vi "Trigger the captured image.vi"() -> ()   [LabVIEW 2009]
uses:
  D/Program Files (x86)/National Instruments/LabVIEW 2015/user.lib/LabViewDVPCamera/LabViewDVPCamera.lvlib
panel:
  in  "Trigger":bool
  in  "CloseFlg":i32
  out "handle":u32
  out "new picture":picture caption="新图片"
  in  "CameraList":u16(ring) items=["USB2_1.2M_MONO(39)@UE121000027", "USB2_3M(19)@1112121"]
  in  "Set":bool
  in  "Close":bool
  in  "Open":bool
  in  "ScanCamera":bool
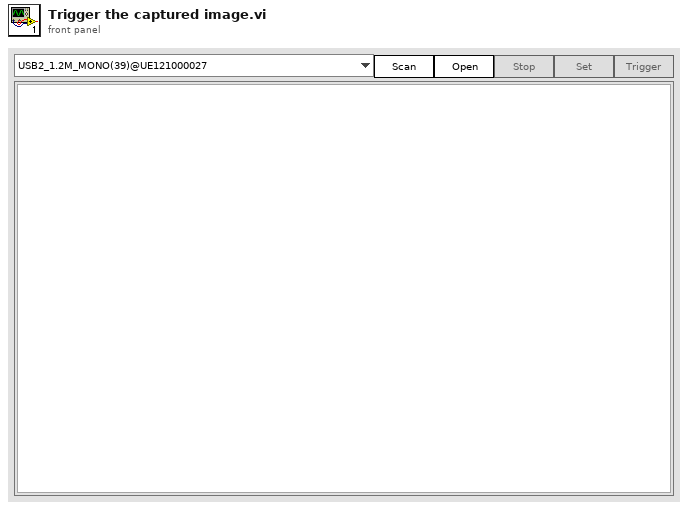
[diagram p1: front panel]
types:
  T1 = enum8{"Enabled", "Disabled", "Disabled and Grayed Out"}
  T2 = typedef "LVStringsAndValuesArrayTypeDef_U16.ctl" = cluster{"String":string, "Value":u16}[]
  T3 = cluster{"image type":i16, "image depth":u8, u8[], "无符号8位数组":u8[], u32[], cluster{u16, u16, u16, u16}}
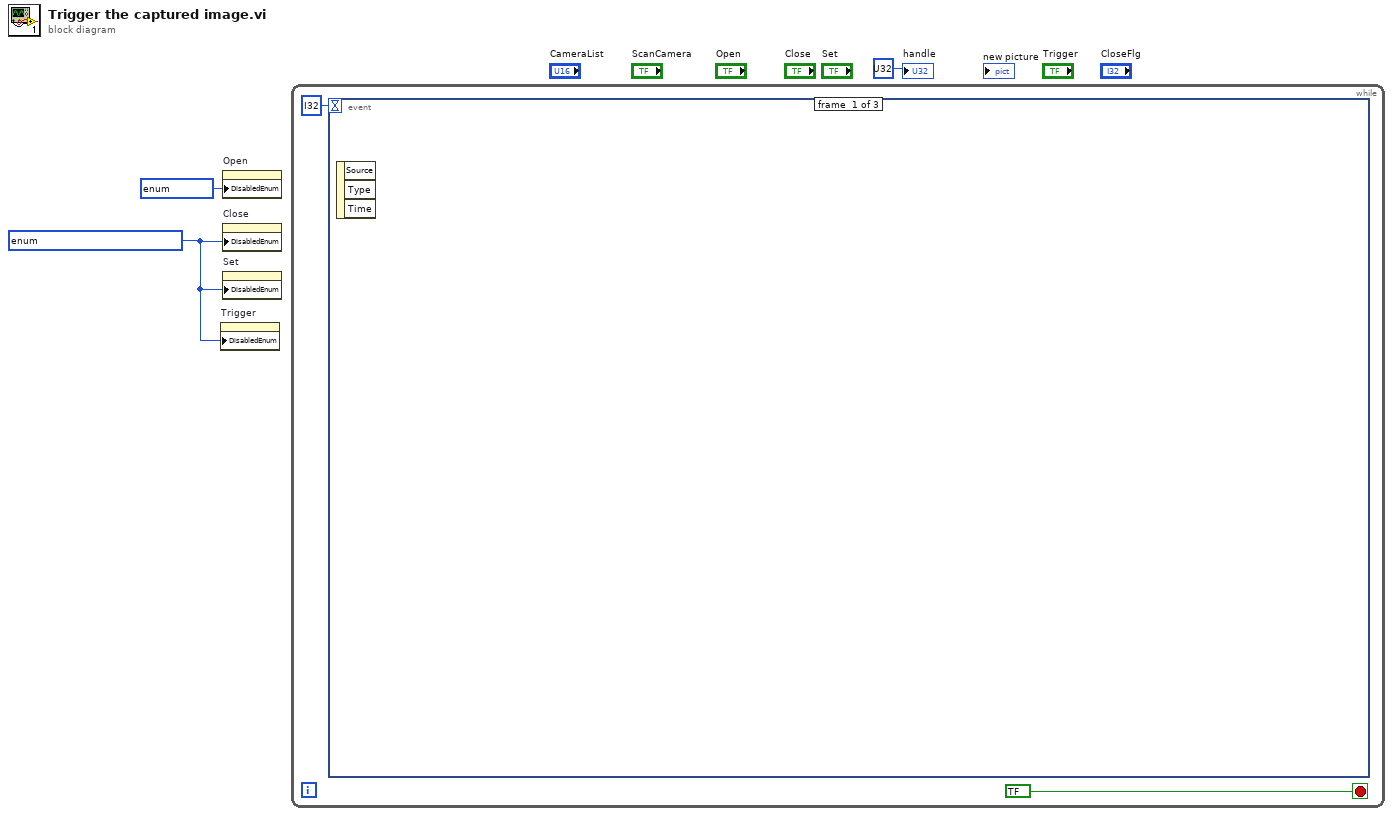
[diagram p0: block diagram]
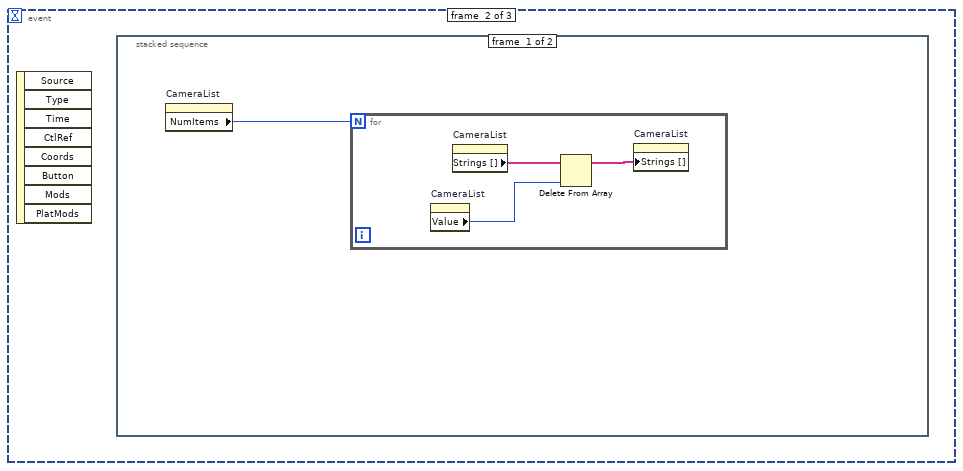
[diagram p2: hidden frame]
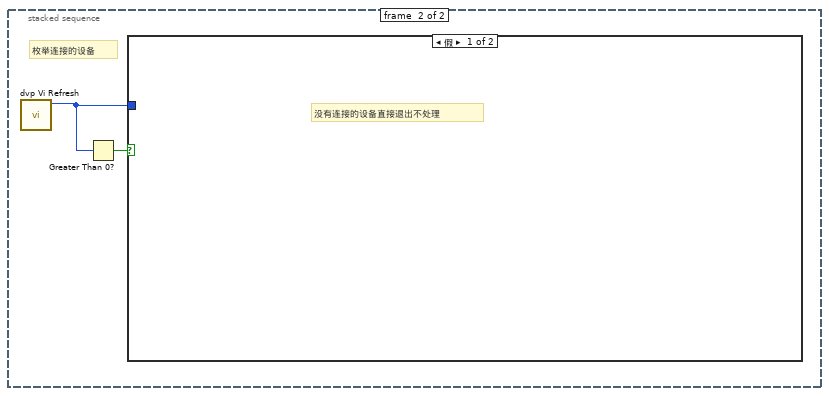
[diagram p3: hidden frame]
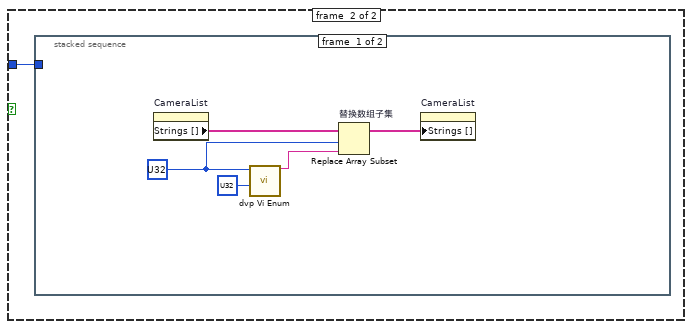
[diagram p4: hidden frame]
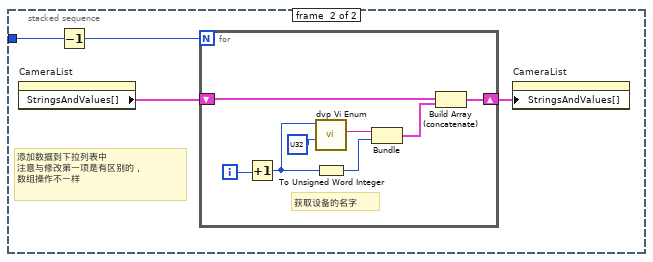
[diagram p5: hidden frame]
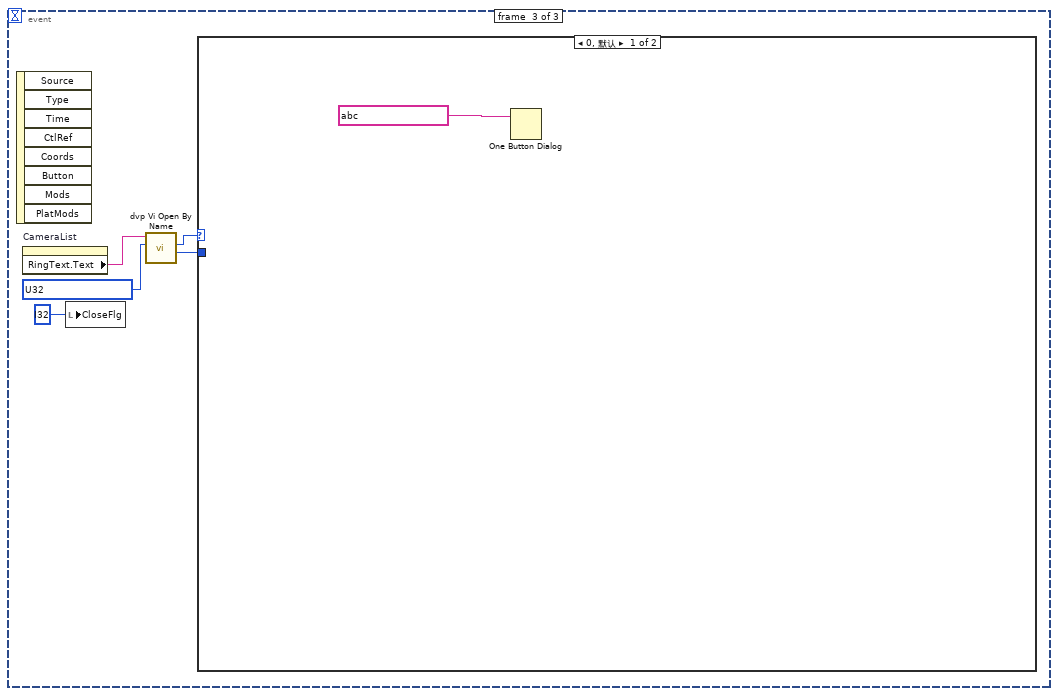
[diagram p6: hidden frame]
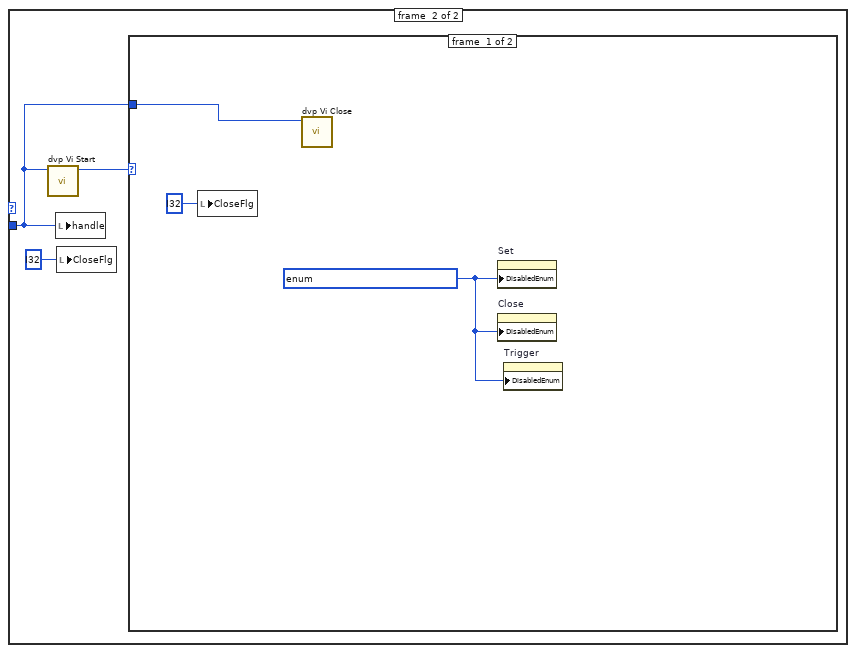
[diagram p7: hidden frame]
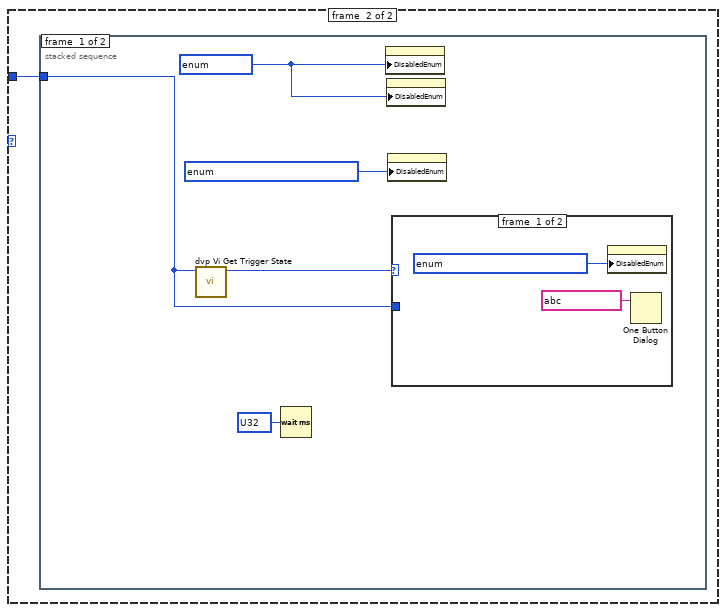
[diagram p8: hidden frame]
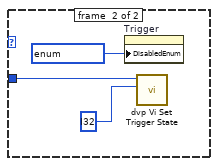
[diagram p9: hidden frame]
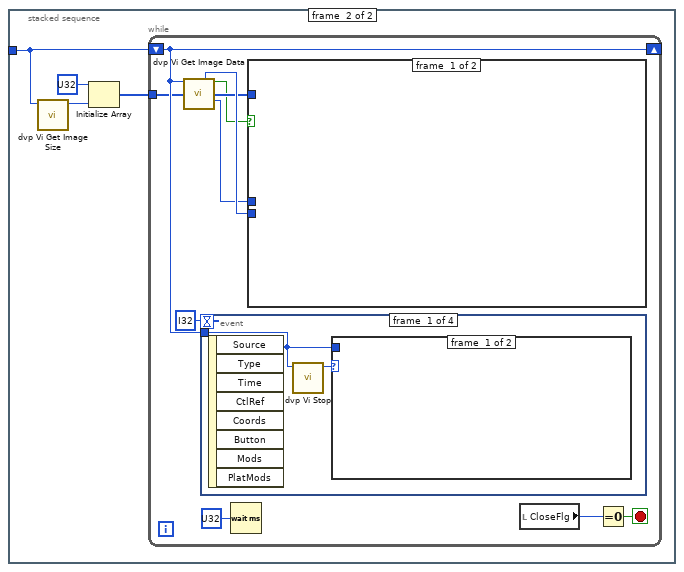
[diagram p10: hidden frame]
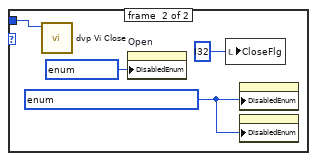
[diagram p11: hidden frame]
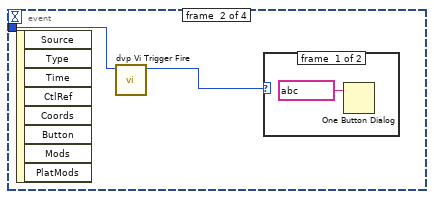
[diagram p12: hidden frame]
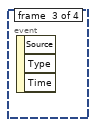
[diagram p14: hidden frame]
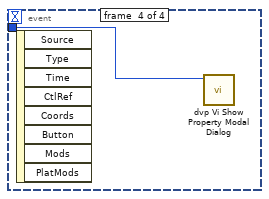
[diagram p15: hidden frame]
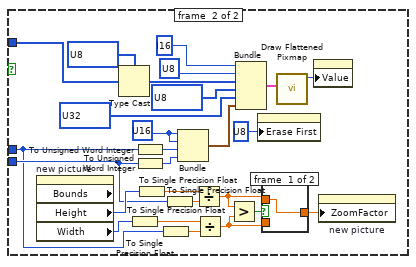
[diagram p16: hidden frame]
diagram:
  w1 = T1 ? ("禁用")
  n1 = property on="Trigger" class="Bool"("DisabledEnum"=w1) -> ()  [unwired: 2 in, 2 out]
  n2 = property on="Open" class="Bool"("DisabledEnum"=T1 ? ("禁用")) -> ()  [unwired: 2 in, 2 out]
  n3 = property on="Close" class="Bool"("DisabledEnum"=w1) -> ()  [unwired: 2 in, 2 out]
  n4 = property on="Set" class="Bool"("DisabledEnum"=w1) -> ()  [unwired: 2 in, 2 out]
  n5 = while {
    stop <- bool ? stop-if-true
    n6 = event shown="[2] \"Open\": 鼠标按下" {
      selector: _ -> [_ _ _]
      dyn-events: _ -> [_ _ _]
      timeout: i32 ? -> [_ _ _]
      event #0 {
        n7 = event-data() -> ()  [unwired: 1 in, 3 out]
      }
      event #1 {
        n8 = event-data() -> ()  [unwired: 1 in, 8 out]
        n9 = stacked-sequence "清除下拉列表的数据" {
          frame #0 {
            n10 = property on="CameraList" class="Ring (严格)"() -> ("NumItems"=w6:u32)  [unwired: 2 in, 2 out]
            n11 = for {
              N: w6 -> [_]
              n12 = property on="CameraList" class="Ring (严格)"() -> ("Value"=w8:u16)  [unwired: 2 in, 2 out]
              n13 = property on="CameraList" class="Ring (严格)"() -> ("Strings []"=w7:string[])  [unwired: 2 in, 2 out]
              n14 = Delete From Array ("删除数组元素")(array=w7, index=w8) -> (array with subset deleted=w9:string[])  [unwired: 1 in, 1 out]
              n15 = property on="CameraList" class="Ring (严格)"("Strings []"=w9) -> ()  [unwired: 2 in, 2 out]
            }
          }
          frame #1 {
            # "枚举连接的设备"
            n16 = call "dvp Vi Refresh.vi"() -> ("pCount out"=w11:u32)  [unwired: 10 in, 1 out]
            n17 = Greater Than 0?(x=w11) -> (x > 0?=w10:bool)
            n18 = case shown="假" w10 {
              tunnel: w11 -> [_ w12]
              frame #0 {
                # "没有连接的设备直接退出不处理"
              }
              frame #1 {
                n19 = stacked-sequence {
                  tunnel: w12 -> [_ w19]
                  frame #0 {
                    w13 = u32 ? ("index")
                    n20 = property on="CameraList" class="Ring (严格)"() -> ("Strings []"=w16:string[])  [unwired: 2 in, 2 out]
                    n21 = call "dvp Vi Enum.vi"("unSize"=u32 ?, "index"=w13) -> ("friendlyName out"=w15:string)  [unwired: 8 in, 1 out]
                    n22 = Replace Array Subset "替换数组子集"(array=w16, new element=w15, index=w13) -> (w17:string[])
                    n23 = property on="CameraList" class="Ring (严格)"("Strings []"=w17) -> ()  [unwired: 2 in, 2 out]
                  }
                  frame #1 {
                    # "添加数据到下拉列表中\n注意与修改第一项是有区别的，\n数组操作不一样"
                    n24 = property on="CameraList" class="Ring (严格)"() -> ("StringsAndValues[]"=w21:T2)  [unwired: 2 in, 2 out]
                    n25 = Decrement(x=w19) -> (x-1=w18:u32)
                    n26 = for {
                      N: w18 -> [_]
                      shift-right: [w28] -> w20
                      shift-left: w21 -> [w26]
                      i -> [w23]
                      # "获取设备的名字"
                      n27 = Increment(x=w23) -> (x+1=w22:i32)
                      n28 = call "dvp Vi Enum.vi"("unSize"=u32 ?, "index"=w22) -> ("friendlyName out"=w29:string)  [unwired: 8 in, 1 out]
                      n29 = To Unsigned Word Integer(number=w22) -> (unsigned 16bit integer=w25:u16)
                      n30 = Bundle("friendlyName out"=w29, w25) -> (w27:cluster{"friendlyName out":string, u16})  [unwired: 1 in]
                      n31 = Build Array (concatenate)(w26, w27) -> (w28:T2)
                    }
                    n32 = property on="CameraList" class="Ring (严格)"("StringsAndValues[]"=w20) -> ()  [unwired: 2 in, 2 out]
                  }
                }
              }
            }
          }
        }
      }
      event #2 {
        w32 = u32 ? items=["OPEN_OFFLINE", "OPEN_NORMAL"] ("type")
        n33 = event-data() -> ()  [unwired: 1 in, 8 out]
        n34 = property on="CameraList" class="Ring (严格)"() -> ("RingText.Text"=w31:string)  [unwired: 2 in, 2 out]
        n35 = local write "CloseFlg"(i32 ? ("CloseFlg")) -> ()
        n36 = call "dvp Vi Open By Name.vi"("type"=w32, "friendlyName"=w31) -> ("pHandle out"=w34:u32, "function return"=w33:u32)  [unwired: 7 in, 1 out]
        n37 = case shown="0, 默认" w33 {
          tunnel: w34 -> [_ w38]
          frame #0 {
            n38 = One Button Dialog(message=string ? ("消息")) -> ()  [unwired: 1 in, 1 out]
          }
          frame #1 {
            n39 = call "dvp Vi Start.vi"("handle"=w38) -> ("function return"=w36:u32)  [unwired: 10 in]
            n40 = local write "handle"(w38) -> ()
            n41 = local write "CloseFlg"(i32 ? ("CloseFlg")) -> ()
            n42 = case shown="1" w36 {
              tunnel: w38 -> [w41 w42]
              frame #0 {
                w39 = T1 ? ("禁用")
                n43 = local write "CloseFlg"(i32 ? ("CloseFlg")) -> ()
                n44 = call "dvp Vi Close.vi"("handle"=w41) -> ()  [unwired: 10 in, 1 out]
                n45 = property on="Set" class="Bool"("DisabledEnum"=w39) -> ()  [unwired: 2 in, 2 out]
                n46 = property on="Close" class="Bool"("DisabledEnum"=w39) -> ()  [unwired: 2 in, 2 out]
                n47 = property on="Trigger" class="Bool"("DisabledEnum"=w39) -> ()  [unwired: 2 in, 2 out]
              }
              frame #1 {
                n48 = stacked-sequence {
                  tunnel: w42 -> [w44 w54]
                  frame #0 {
                    w46 = T1 ? ("禁用")
                    n49 = call "dvp Vi Get Trigger State.vi"("handle"=w44) -> ("function return"=w45:u32)  [unwired: 9 in, 1 out]
                    n50 = Wait (ms)(milliseconds to wait=u32 ? ("等待时间（毫秒）")) -> ()  [unwired: 1 out]
                    n51 = property on="Set" class="Bool"("DisabledEnum"=w46) -> ()  [unwired: 2 in, 2 out]
                    n52 = property on="Close" class="Bool"("DisabledEnum"=w46) -> ()  [unwired: 2 in, 2 out]
                    n53 = property on="Open" class="Bool"("DisabledEnum"=T1 ? ("禁用")) -> ()  [unwired: 2 in, 2 out]
                    n54 = case shown="1" w45 {
                      tunnel: w44 -> [_ w51]
                      frame #0 {
                        n55 = property on="Trigger" class="Bool"("DisabledEnum"=T1 ? ("禁用")) -> ()  [unwired: 2 in, 2 out]
                        n56 = One Button Dialog(message=string ? ("消息")) -> ()  [unwired: 1 in, 1 out]
                      }
                      frame #1 {
                        n57 = property on="Trigger" class="Bool"("DisabledEnum"=T1 ? ("禁用")) -> ()  [unwired: 2 in, 2 out]
                        n58 = call "dvp Vi Set Trigger State.vi"("TriggerState"=i32 ?, "handle"=w51) -> ()  [unwired: 9 in, 1 out]
                      }
                    }
                  }
                  frame #1 {
                    n59 = call "dvp Vi Get Image Size.vi"("handle"=w54) -> ("function return"=w55:u32)  [unwired: 10 in]
                    n60 = Initialize Array(u32 ? ("元素"), w55) -> (w53:u32[])
                    n61 = while {
                      shift-right: [w62] -> _
                      shift-left: w54 -> [w62]
                      tunnel: w53 -> [w61]
                      stop <- w65 stop-if-true
                      n62 = call "dvp Vi Get Image Data.vi"("handle"=w62, "pbuffer"=w61) -> ("piHeight out"=w60:i32, "function return"=w57:bool, "pbuffer out"=w58:u32[], "piWidth out"=w59:i32)  [unwired: 9 in, 1 out]
                      n63 = event shown="[3] \"Set\": 鼠标按下" {
                        selector: _ -> [_ _ _ _]
                        dyn-events: _ -> [_ _ _ _]
                        timeout: i32 ? -> [_ _ _ _]
                        tunnel: w62 -> [w67 w74 _ w76]
                        event #0 {
                          n64 = event-data() -> ()  [unwired: 1 in, 8 out]
                          n65 = call "dvp Vi Stop.vi"("handle"=w67) -> ("function return"=w68:u32)  [unwired: 10 in]
                          n66 = case shown="1" w68 {
                            tunnel: w67 -> [_ w70]
                            frame #0 {
                            }
                            frame #1 {
                              w69 = T1 ? ("禁用")
                              n67 = call "dvp Vi Close.vi"("handle"=w70) -> ()  [unwired: 10 in, 1 out]
                              n68 = property on="Open" class="Bool"("DisabledEnum"=T1 ? ("禁用")) -> ()  [unwired: 2 in, 2 out]
                              n69 = local write "CloseFlg"(i32 ? ("CloseFlg")) -> ()
                              n70 = property on="Close" class="Bool"("DisabledEnum"=w69) -> ()  [unwired: 2 in, 2 out]
                              n71 = property on="Set" class="Bool"("DisabledEnum"=w69) -> ()  [unwired: 2 in, 2 out]
                            }
                          }
                        }
                        event #1 {
                          n72 = event-data() -> ()  [unwired: 1 in, 8 out]
                          n73 = call "dvp Vi Trigger Fire.vi"("handle"=w74) -> ("function return"=w73:u32)  [unwired: 10 in]
                          n74 = case shown="1" w73 {
                            frame #0 {
                              n75 = One Button Dialog(message=string ? ("消息")) -> ()  [unwired: 1 in, 1 out]
                            }
                            frame #1 {
                            }
                          }
                        }
                        event #2 {
                          n76 = event-data() -> ()  [unwired: 1 in, 3 out]
                        }
                        event #3 {
                          n77 = event-data() -> ()  [unwired: 1 in, 8 out]
                          n78 = call "dvp Vi Show Property Modal Dialog.vi"("handle"=w76) -> ()  [unwired: 10 in, 1 out]
                        }
                      }
                      n79 = Wait (ms)(milliseconds to wait=u32 ? ("等待时间（毫秒）")) -> ()  [unwired: 1 out]
                      n80 = case shown="真" w57 {
                        tunnel: w59 -> [_ w77]
                        tunnel: w60 -> [_ w78]
                        tunnel: w58 -> [_ w79]
                        frame #0 {
                        }
                        frame #1 {
                          w99 = u16 ?
                          n81 = property on="new picture" class="Pict" props=[]() -> ("Height"=w94:u32, "Width"=w93:u32)  [unwired: 2 in, 3 out]
                          n82 = Type Cast(type=u8[] ?, x=w79) -> (*(type *) &x=w83:u8[])
                          n83 = To Single Precision Float(number=w93) -> (single precision float=w86:sgl)
                          n84 = To Unsigned Word Integer(number=w77) -> (unsigned 16bit integer=w98:u16)
                          n85 = To Unsigned Word Integer(number=w78) -> (unsigned 16bit integer=w97:u16)
                          n86 = To Single Precision Float(number=w94) -> (single precision float=w92:sgl)
                          n87 = To Single Precision Float(number=w77) -> (single precision float=w90:sgl)
                          n88 = To Single Precision Float(number=w78) -> (single precision float=w91:sgl)
                          n89 = Bundle ("图像尺寸")(w99, w99, w98, w97) -> (w96:cluster{u16, u16, u16, u16})  [unwired: 1 in]
                          n90 = Divide(x=w92, y=w91) -> (x/y=w88:sgl)
                          n91 = Divide(x=w86, y=w90) -> (x/y=w87:sgl)
                          n92 = Greater?(x=w88, y=w87) -> (0:w89:bool)
                          n93 = Bundle ("图像数据")("image type"=i16 ?, "image depth"=u8 ?, w83, "无符号8位数组"=u8[] ?, u32[] ?, w96) -> (w84:T3)  [unwired: 1 in]
                          n94 = property on="new picture" class="Pict"("Erase First"=u8 ? ("画前清除图片")) -> ()  [unwired: 2 in, 2 out]
                          n95 = case shown="真" w89 {
                            tunnel: w88 -> [w103 _]
                            tunnel: w87 -> [_ w104]
                            tunnel: [w103 w104] -> w85
                            frame #0 {
                            }
                            frame #1 {
                            }
                          }
                          n96 = call <vilib>:"Draw Flattened Pixmap.vi"("image data"=w84) -> ("new picture"=w80:picture)  [unwired: 8 in]
                          n97 = property on="new picture" class="Pict"("Value"=w80) -> ()  [unwired: 2 in, 2 out]
                          n98 = property on="new picture" class="Pict"("ZoomFactor"=w85) -> ()  [unwired: 2 in, 2 out]
                        }
                      }
                      n99 = local read "CloseFlg"() -> (w64:i32)
                      n100 = Equal To 0?(x=w64) -> (x = 0?=w65:bool)
                    }
                  }
                }
              }
            }
          }
        }
      }
    }
  }
  "handle" <- u32 ? ("handle")
